vi "niRFUtil RFHS Benchmark Leave.vi"(7 "Skip":bool, 9 "error in (no error)":errorcluster, 11 "Benchmark Task Self":T1) -> (1 "error out":errorcluster, 3 "Benchmark Task Owner":T1)   [LabVIEW 2015, in "niRFUtil.lvlib"]
uses:
  niRFUtil.lvlib
  niRFUtil RFHS Benchmark Task.ctl
  niRFUtil RFHS Util Phases.ctl
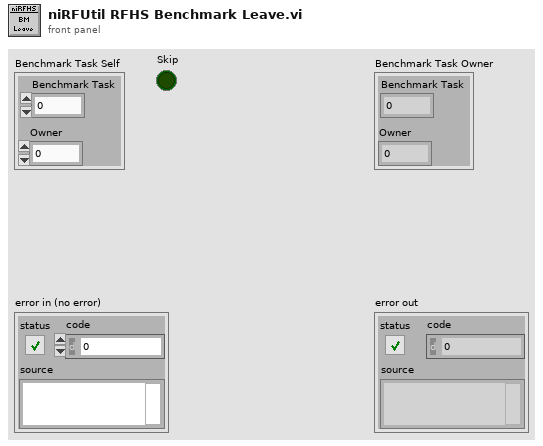
[diagram p1: front panel]
types:
  T1 = typedef "niRFUtil.lvlib/niRFUtil RFHS Benchmark Task.ctl" = cluster{"Benchmark Task":u64, "Owner":u32}
  T2 = typedef "niRFUtil.lvlib/niRFUtil RFHS Util Phases.ctl" = enum32{"Reserved", "CreateBenchmarkTask", "CRC", "UE UL Segment Transport Block", "UE UL Read Buffer", "UE UL TC", "UE UL RM", "UE UL CI", "Scramble", "Group Bits", "Benchmark Task Start", "Benchmark Task Stop", "Descramble", "Deinterleave", "eNB UL HARQ", "eNB UL Read Buffer", "eNB UL AFEM", "eNB UL Turbo Decoder", "Get Benchmark Task Data", "G31", "UL Gen Freq2Time", "Gen Power Spectrum", "UL Ana Time2Freq", "Benchmark Task Enter", "Benchmark Task Leave"}
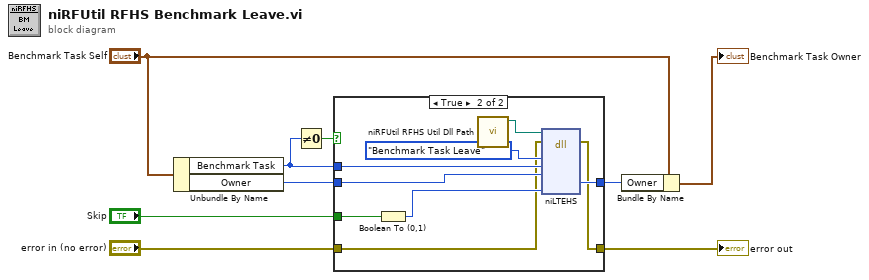
[diagram p0: block diagram]
diagram:
  n1 = Unbundle By Name("Benchmark Task Self") -> ("Benchmark Task"=w3:u64, "Owner"=w9:u32)
  n2 = Not Equal To 0?(x=w3) -> (x != 0?=w5:bool)
  n3 = case shown="True" w5 {
    tunnel: w3 -> [_ w18]
    tunnel: w9 -> [w11 w17]
    tunnel: [w11 w16] -> w7
    tunnel: "Skip" -> [_ w15]
    tunnel: [w10 w13] -> w2
    tunnel: "error in (no error)" -> [w10 w12]
    frame False {
    }
    frame True {
      n4 = Boolean To (0,1)(Boolean=w15) -> (0, 1=w14:i16)
      n5 = call "niRFUtil RFHS Util Dll Path.vi"() -> ("Path"=w20:path)  [unwired: 7 in, 4 out]
      n6 = dll-call lib="C:/ni-rt/system/HPCExecBenchDll.dll" fn="niLTEHS"(path in=w20, error in=w12, "what"=niRFUtil_RFHS_Util_Phases."Benchmark Task Leave" ("Enum"), "benchmarkTask"=w18, "benchId"=w17, "skip"=w14) -> (error out=w13:errorcluster, "owner"=w16:u32)  [unwired: 7 in, 1 out]
    }
  }
  "error out" <- w2
  n7 = Bundle By Name(cluster="Benchmark Task Self", "Owner"=w7) -> (→"Benchmark Task Owner":T1)
